vi "Get Data.vi"(11 "Persistent Path Selector in":refnum<class "MGI Persistent Path Selector.lvclass">) -> (2 "Persistent":T1={"Initial Path"=path "", "INI Path"=path "", "INI Section"="Last Used", "Select Option?"=TRUE, "Explorer Option?"=TRUE, "Recurse?"=TRUE, "Allow New?"=FALSE, "Filter"="*.*"})   [LabVIEW 2016, in "MGI Persistent Path Selector.lvclass"]
doc: "Set protected data."
uses:
  <userlib>/_MGI/User Interface/Path Selector XControl/Class Hierarchy/Persistent Path Selector/MGI Persistent Path Selector.lvclass
  <userlib>/_MGI/User Interface/Path Selector XControl/Class Hierarchy/Persistent Path Selector/Persistent Data Cluster.ctl
  <userlib>/_MGI/User Interface/Path Selector XControl/Class Hierarchy/Persistent Path Selector/MGI Persistent Path Selector.lvclass/MGI Persistent Path Selector.ctl
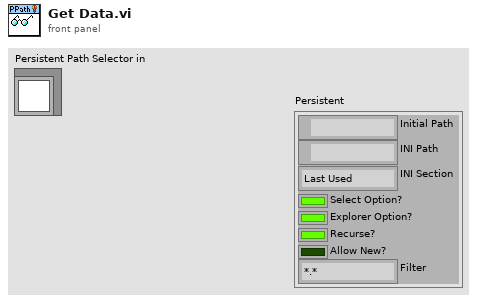
[diagram p1: front panel]
types:
  T1 = typedef "MGI Persistent Path Selector.lvclass/Persistent Data Cluster.ctl" = cluster{"Initial Path":path, "INI Path":path, "INI Section":string, "Select Option?":bool, "Explorer Option?":bool, "Recurse?":bool, "Allow New?":bool, "Filter":string}
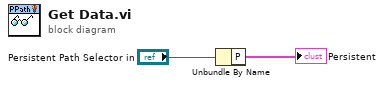
[diagram p0: block diagram]
diagram:
  n1 = Unbundle By Name("Persistent Path Selector in") -> ("P"=→"Persistent":T1)
